vi "Error to Warning.vi"(7 "Change to warning?":bool, 11 "error in (no error)":errorcluster) -> (3 "error out":errorcluster)   [LabVIEW 2020]
doc: "Change error to warning, if enabled."
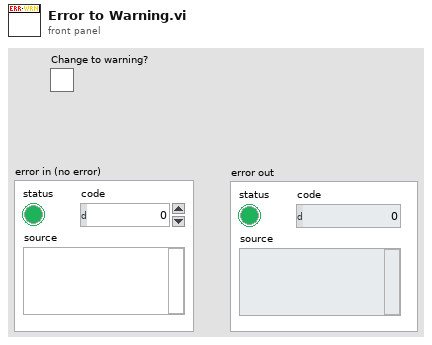
[diagram p1: front panel]
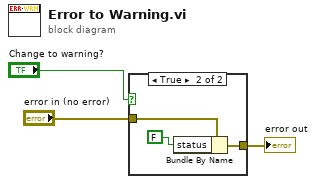
[diagram p0: block diagram]
diagram:
  n1 = case shown="True" "Change to warning?" {
    tunnel: [w4 w7] -> w3
    tunnel: "error in (no error)" -> [w4 w6]
    frame False {
    }
    frame True {
      n2 = Bundle By Name(cluster=w6, "status"=FALSE) -> (w7:errorcluster)
    }
  }
  "error out" <- w3
